vi "startContinuous.vi"(7 "stop_variable":u8, 8 "error in":errorcluster, 9 "period_ms":u32, 10 "Slave Address(7 bit)":u8, 11 "I2C Ref In":T1) -> (0 "error out":errorcluster, 3 "I2C Ref Out":T1)   [LabVIEW 2018]
uses:
  <vilib>/myRIO/Instrument Drivers/Onboard IO/I2C/typedefs/I2C Reference.ctl
  <vilib>/myRIO/Common/Instrument Driver Framework/Utilities/typedefs/myRIO Generic Hardware Reference.ctl
  <vilib>/myRIO/Common/Instrument Driver Framework/Utilities/typedefs/Hardware Version Enum.ctl
  <vilib>/myRIO/Common/Instrument Driver Framework/Utilities/typedefs/myRIO v1.0 Reference.ctl
  <vilib>/myRIO/Common/Instrument Driver Framework/Utilities/typedefs/Generic FPGA Reference.ctl
  <vilib>/myRIO/Common/Instrument Driver Framework/myRIO v1.0/I2C/typedefs/I2C Channels Enum.ctl
  <vilib>/myRIO/Instrument Drivers/Onboard IO/I2C/typedefs/I2C Configuration.ctl
  <vilib>/myRIO/Instrument Drivers/Onboard IO/I2C/typedefs/I2C Transfer Rate.ctl
  <vilib>/Utility/error.llb/Error Cluster From Error Code.vi
  <vilib>/myRIO/Common/Instrument Driver Framework/myRIO v1.0/I2C/vis/myRIO v1.0 Write I2C.vi
  <vilib>/myRIO/Common/Instrument Driver Framework/myRIO v1.0/I2C/vis/myRIO v1.0 Read I2C.vi
  <vilib>/myRIO/Instrument Drivers/Onboard IO/I2C/I2C.lvlib
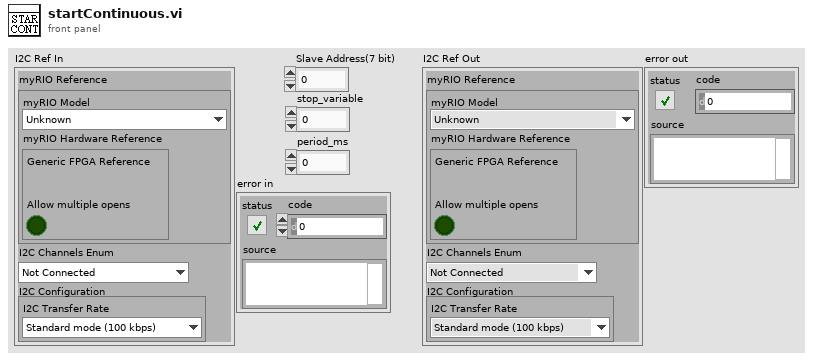
[diagram p1: front panel]
types:
  T1 = typedef "I2C.lvlib/I2C Reference.ctl" = cluster{"myRIO Reference":T2, "I2C Channels Enum":T6, "I2C Configuration":T7}
  T2 = typedef "myRIO Generic Hardware Reference.ctl" = cluster{"myRIO Model":T3, "myRIO Hardware Reference":T4}
  T3 = typedef "Hardware Version Enum.ctl" = enum16{"Unknown", "myRIO-1900", "myRIO-1950", "roboRIO", "NI ELVIS RIO CM", "ELVIS III"}
  T4 = typedef "myRIO v1.0 Reference.ctl" = cluster{"Generic FPGA Reference":T5, "Allow multiple opens":bool}
  T5 = typedef "Generic FPGA Reference.ctl" = refnum<k20>
  T6 = typedef "I2C Channels Enum.ctl" = enum16{"Not Connected", "A/I2C", "B/I2C", "I2C/I2C"}
  T7 = typedef "I2C.lvlib/I2C Configuration.ctl" = cluster{"I2C Transfer Rate":T8}
  T8 = typedef "I2C.lvlib/I2C Transfer Rate.ctl" = enum16{"Standard mode (100 kbps)", "Fast mode (400 kbps)"}
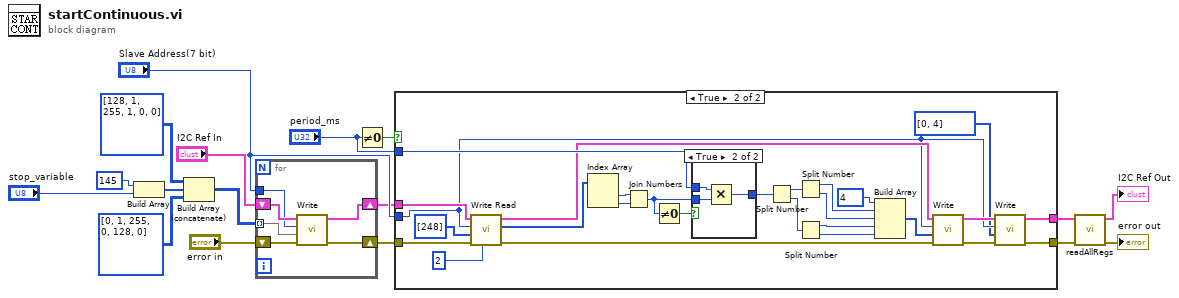
[diagram p0: block diagram]
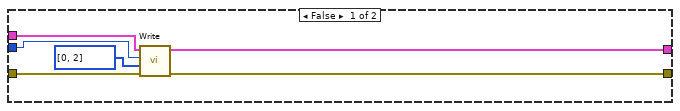
[diagram p2: hidden frame]
diagram:
  n1 = Build Array(u8 145, "stop_variable") -> (w10:u8[])
  n2 = Build Array (concatenate)(u8[][] [[128, 1], [255, 1], [0, 0]] ("Bytes to Write"), w10, u8[][] [[0, 1], [255, 0], [128, 0]] ("Bytes to Write")) -> (w13:u8[][])
  n3 = for {
    tunnel: w13 -> [w23] mode=indexing
    shift-right: [w19] -> w6
    shift-left: "I2C Ref In" -> [w22]
    shift-right: [w20] -> w5
    shift-left: "error in" -> [w21]
    tunnel: "Slave Address(7 bit)" -> [w18]
    n4 = call <vilib>:"Write.vi"("error in (no error)"=w21, "Bytes to Write"=w23, "Slave Address (7-bit)"=w18, "I2C Ref In"=w22) -> ("error out"=w20:errorcluster, "I2C Ref Out"=w19:T1)  [unwired: 6 in]
  }
  n5 = Not Equal To 0?(x="period_ms") -> (x != 0?=w14:bool)
  n6 = case shown="True" w14 {
    tunnel: w6 -> [w28 w54]
    tunnel: w5 -> [w27 w53]
    tunnel: "Slave Address(7 bit)" -> [w24 w33]
    tunnel: "period_ms" -> [_ w48]
    tunnel: [w26 w31] -> w4
    tunnel: [w25 w30] -> w3
    frame False {
      n7 = call <vilib>:"Write.vi"("error in (no error)"=w27, "Bytes to Write"=u8[] [0, 2], "Slave Address (7-bit)"=w24, "I2C Ref In"=w28) -> ("error out"=w25:errorcluster, "I2C Ref Out"=w26:T1)  [unwired: 6 in]
    }
    frame True {
      n8 = call <vilib>:"Write Read.vi"("Byte Count"=u32 2, "error in (no error)"=w53, "Bytes to Write"=u8[] [248], "Slave Address (7-bit)"=w33, "I2C Ref In"=w54) -> ("error out"=w37:errorcluster, "Bytes Read"=w51:u8[], "I2C Ref Out"=w38:T1)  [unwired: 3 in]
      n9 = Index Array(array=w51) -> (element #1=w49:u8, element #2=w50:u8)  [unwired: 2 in]
      n10 = Join Numbers(hi=w49, lo=w50) -> ((hi.lo)=w47:u16)
      n11 = Not Equal To 0?(x=w47) -> (x != 0?=w52:bool)
      n12 = case shown="True" w52 {
        tunnel: w48 -> [w57 w60]
        tunnel: w47 -> [_ w59]
        tunnel: [w57 w58] -> w43
        frame False {
        }
        frame True {
          n13 = Multiply(x=w60, y=w59) -> (x*y=w58:u32)
        }
      }
      n14 = Split Number(x=w43) -> (hi(x)=w45:u16, lo(x)=w44:u16)
      n15 = Split Number(x=w45) -> (hi(x)=w42:u8, lo(x)=w41:u8)
      n16 = Split Number(x=w44) -> (hi(x)=w40:u8, lo(x)=w39:u8)
      n17 = Build Array(u8 4, w42, w41, w40, w39) -> (w36:u8[])
      n18 = call <vilib>:"Write.vi"("error in (no error)"=w37, "Bytes to Write"=w36, "Slave Address (7-bit)"=w33, "I2C Ref In"=w38) -> ("error out"=w34:errorcluster, "I2C Ref Out"=w35:T1)  [unwired: 6 in]
      n19 = call <vilib>:"Write.vi"("error in (no error)"=w34, "Bytes to Write"=u8[] [0, 4], "Slave Address (7-bit)"=w33, "I2C Ref In"=w35) -> ("error out"=w30:errorcluster, "I2C Ref Out"=w31:T1)  [unwired: 6 in]
    }
  }
  n20 = call "readAllRegs.vi"("error in"=w3, "I2C Ref In"=w4) -> ("error out"=→"error out":errorcluster, "I2C Ref Out"=→"I2C Ref Out":T1)  [unwired: 6 in, 2 out]
